vi "Create Stat Array.vi"(0 "DataIn":string[][](array[string]), 11 "Indexes":i32[](array[numeric])) -> (8 "StatArray":string[][](array[string]))   [LabVIEW 2013]
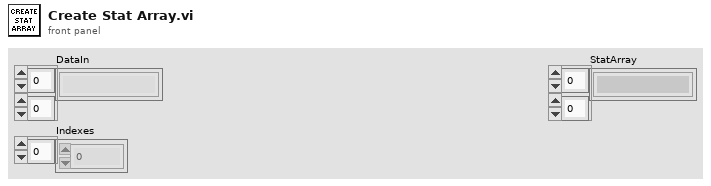
[diagram p1: front panel]
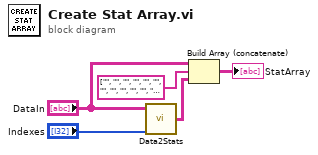
[diagram p0: block diagram]
diagram:
  n1 = call "Data2Stats.vi"("DataIn"="DataIn", "Indexes"="Indexes") -> ("StatsOut"=w4:string[][])  [unwired: 13 in]
  n2 = Build Array (concatenate)("DataIn", string[] ["", "", "", "", "", "", "", "", "", "", "", "", "", ""], w4) -> (→"StatArray":string[][])
